vi "Imagen_3D.vi"() -> ()   [LabVIEW 2016]
uses:
  <vilib>/Utility/miscctls.llb/LV3DPointTypeDef.ctl
  <vilib>/picture/3D Picture Control/NI_3D Picture Control.lvlib
panel:
  in  "Stop Button":bool
  in  "Up Direction":T1
  in  "Target":T1
  in  "Camera Position":T1
  out "3D Picture":refnum<vi>(3d-picture)
  in  "Path":path
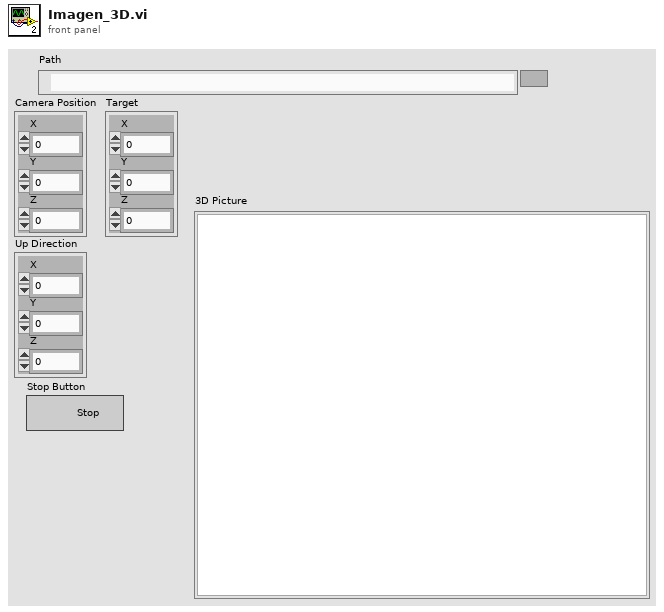
[diagram p1: front panel]
types:
  T1 = typedef "LV3DPointTypeDef.ctl" = cluster{"X":sgl, "Y":sgl, "Z":sgl}
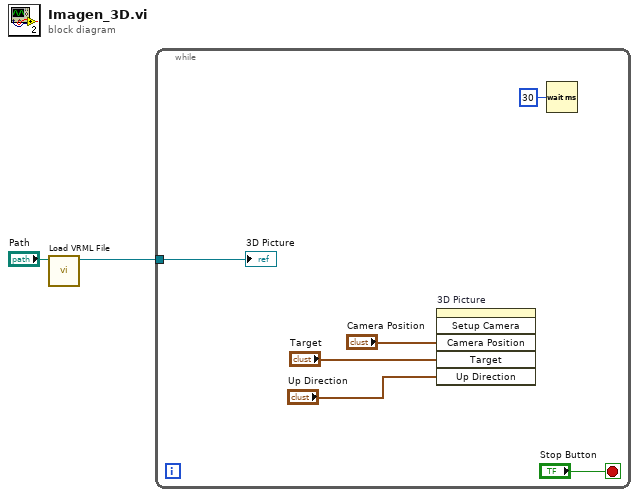
[diagram p0: block diagram]
diagram:
  n1 = call <vilib>:"Load VRML File.vi"("Path"="Path") -> ("Scene:Read Scene File"=w1:refnum<vi>)  [unwired: 9 in, 1 out]
  n2 = while {
    tunnel: w1 -> [w7]
    stop <- "Stop Button" stop-if-true
    n3 = invoke on="3D Picture" class="SceneGraphDisp (strict)" method="Setup Camera"("Camera Position"="Camera Position", "Target"="Target", "Up Direction"="Up Direction") -> ()  [unwired: 3 in, 6 out]
    n4 = Wait (ms)(milliseconds to wait=u32 30) -> ()  [unwired: 1 out]
    "3D Picture" <- w7
  }
